vi "Start Run.vi"(8 "error in (no error)":errorcluster, 11 "DAQ Manager in":refnum<class "DAQ Manager.lvclass">) -> (0 "error out":errorcluster, 1 "TCP Port Number":u32, 2 "Run Number":u32, 3 "DAQ Manager out":refnum<class "DAQ Manager.lvclass">, 4 "Data storage path":string, 5 "Run Active?":bool)   [LabVIEW 2020, in "DAQ Manager.lvlib" / "DAQ Manager.lvclass"]
uses:
  DAQ Manager.lvclass
  DAQ Manager.lvclass/DAQ Manager.ctl
  Ancestor/Ancestor/Ancestor.lvclass/Ancestor.ctl
  Support VIs/Generate Error.vi
  FGV/Error Memory/Get Error Description.vi
  Support VIs/Get PC name.vi
  Ancestor/Ancestor/Read ID.vi
  Support VIs/Get Class Name.vi
  <vilib>/Utility/error.llb/Clear Errors.vi
  FGV/Error Memory/Error Memory Core.vi
  <vilib>/AdvancedString/Delimited String to 1D String Array.vi
  Support VIs/Circus Root Path.vi
  FGV/Error Memory/Error Crt Lvl checker.vi
  FGV/Error Memory/Error Memory Core.vi/40c8088d-b597-4017-91af-faa98e00292e.vi
  FGV/Error Memory/Error Memory Core.vi/d4a3ab98-063c-4e44-b43d-fbdcfe6c2be2.vi
  Support VIs/Global Memory.vi
  <vilib>/Utility/LVClass/Get LV Class Name.vi
  Support VIs/Is in Packed Library.vi
  Support VIs/TALOS Root path.vi
  Support VIs/Read CSV worksheet.vi
  Support VIs/Global Constants.vi
  <vilib>/Utility/error.llb/General Error Handler.vi
  Support VIs/Error Log.vi
  Ancestor/Ancestor/Ancestor.lvclass
  <vilib>/Comparison/Equal/Equal Functor/Equal Functor.lvclass
  Interfaces/DAQ Control/DAQ Control.lvclass
  TALOS.lvlib
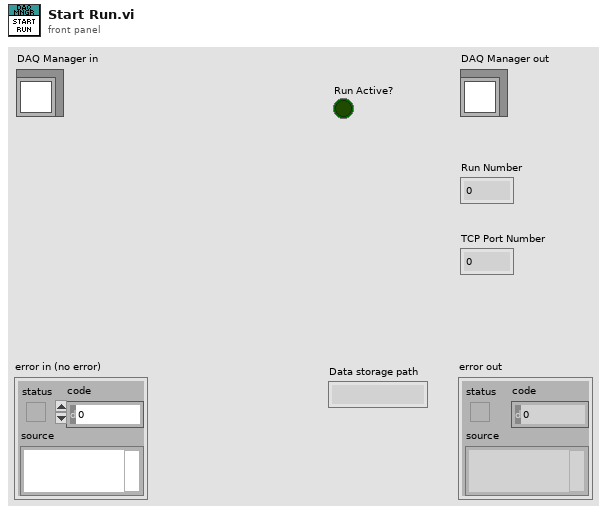
[diagram p1: front panel]
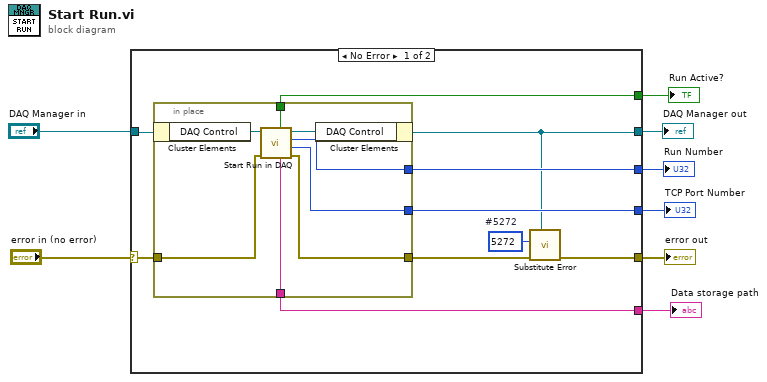
[diagram p0: block diagram]
diagram:
  n1 = case shown="No Error" "error in (no error)" {
    selector: "error in (no error)" -> [w17 w28]
    tunnel: [w11 w28] -> w7
    tunnel: [w10 w27] -> w5
    tunnel: "DAQ Manager in" -> [w18 w27]
    tunnel: [w16 _] -> w4
    tunnel: [w15 _] -> w3
    tunnel: [w14 _] -> w2
    tunnel: [w13 _] -> w1
    frame No Error {
      w9 = 5272  # #5272
      n2 = in-place {
        in-place-border: w17 -> [w24]
        in-place-border: [w23] -> w12
        in-place-border: [w22] -> w16
        in-place-border: [w21] -> w15
        in-place-border: [w20] -> w14
        in-place-border: [w19] -> w13
        n3 = in-place-cluster #1(w18) -> ("DAQ Control"=w26:refnum<class "DAQ Control.lvclass">)
        n4 = call-dynamic "Start Run in DAQ.vi"("error in (no error)"=w24, "DAQ Control in"=w26) -> ("error out"=w23:errorcluster, "TCP Port Number"=w20:u32, "Run Number"=w22:u32, "DAQ Control out"=w25:refnum<class "DAQ Control.lvclass">, "Data storage path"=w19:string, "Run Active?"=w21:bool)  [unwired: 4 in]
        n5 = in-place-cluster #1("DAQ Control"=w25) -> (w10:refnum<class "DAQ Manager.lvclass">)
      }
      n6 = call "Substitute Error.vi"("LabVIEW Object"=w10, "error in (no error)"=w12, "Error Code"=w9) -> ("error out"=w11:errorcluster)  [unwired: 8 in]
    }
    frame Error {
    }
  }
  "error out" <- w7
  "DAQ Manager out" <- w5
  "Run Number" <- w4
  "Run Active?" <- w3
  "TCP Port Number" <- w2
  "Data storage path" <- w1
